vi "temperature_logger_server.vi"(9 "date string":string, 10 "time string":string, 11 "Numeric":dbl) -> ()   [LabVIEW 2017]
uses:
  <vilib>/Utility/file.llb/Write Delimited Spreadsheet (string).vi
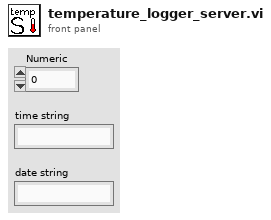
[diagram p1: front panel]
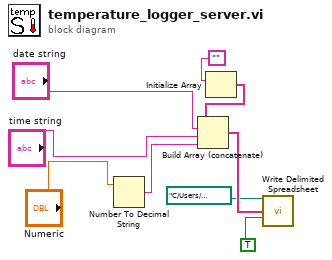
[diagram p0: block diagram]
diagram:
  n1 = Number To Decimal String(number="Numeric") -> (decimal integer string=w5:string)  [unwired: 1 in]
  n2 = Initialize Array("") -> (w8:string[])  [unwired: 1 in]
  n3 = Build Array (concatenate)(w8, "date string", "time string", w5) -> (w9:string[])
  n4 = call-poly <vilib>:"Write Delimited Spreadsheet.vi"("file path (dialog if empty)"=path "C:/Users/Whistleblower/greenfox/Gabor11/week-11/day_04/temp_log.txt", "1D data"=w9, "append to file? (new file:F)"=TRUE) -> ()  [unwired: 11 in, 2 out]
